vi "Write Client Port.vi"(8 "error in (no error)":errorcluster, 10 "Client Port":u16=515, 11 "Event_Syslog in":refnum<class "Event_Syslog.lvclass">) -> (0 "error out":errorcluster, 3 "Event_Syslog out":refnum<class "Event_Syslog.lvclass">)   [LabVIEW 2021, in "Event_Syslog.lvclass"]
uses:
  Event_Syslog.lvclass
  Event_Syslog.lvclass/Event_Syslog.ctl
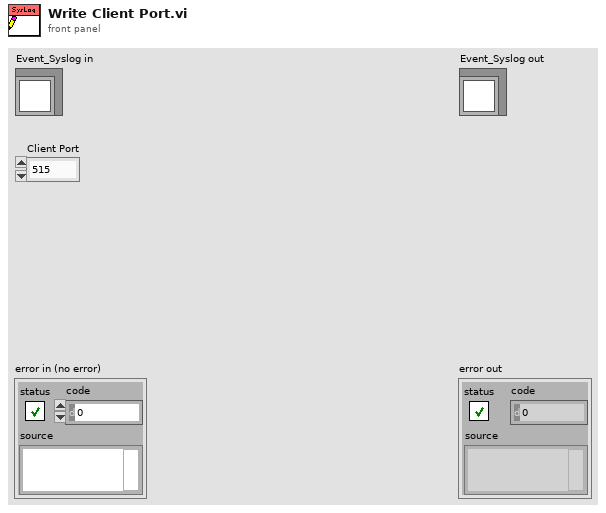
[diagram p1: front panel]
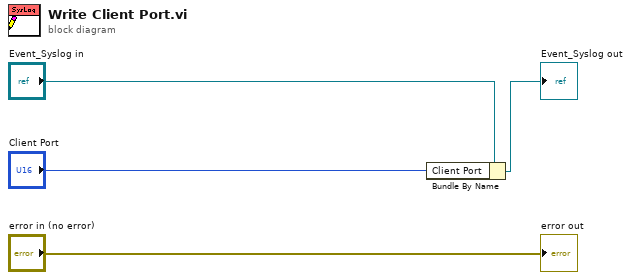
[diagram p0: block diagram]
diagram:
  n1 = Bundle By Name(cluster="Event_Syslog in", "Client Port"="Client Port") -> (→"Event_Syslog out":refnum<class "Event_Syslog.lvclass">)
  "error out" <- "error in (no error)"
